vi "NTCP Read Msgs.vi"(5 "NTCP Read In":refnum<queue>, 7 "NTCP send in":refnum<queue>, 8 "error in (no error)":errorcluster, 11 "NTCP Actions":T4) -> (0 "error out":errorcluster, 1 "Targets":T2[](array[typedef]), 2 "Transaction ID":string, 3 "NTCP Status":T1, 4 "NTCP Read Out":refnum<queue>, 6 "NTCP send out":refnum<queue>)   [LabVIEW 2009]
uses:
  Launcher/Launcher Actions.ctl
  Launcher/NoPanelAppTypes.ctl
  Apps/App Status Actions.ctl
  NTCP library/NTCP Commands.ctl
  Data Access Objects/Metadata/LBCB Number.ctl
  MixedMode/Widget/Target.ctl
  NTCP Msg Types.ctl
  Global Data/Cartesian Measurment Actions.ctl
  NTCP Status.ctl
  Control Point Suffix.ctl
  NTCP library/Payload.ctl
  NTCP library/NTCP Message.ctl
  NTCP Client Actions.ctl
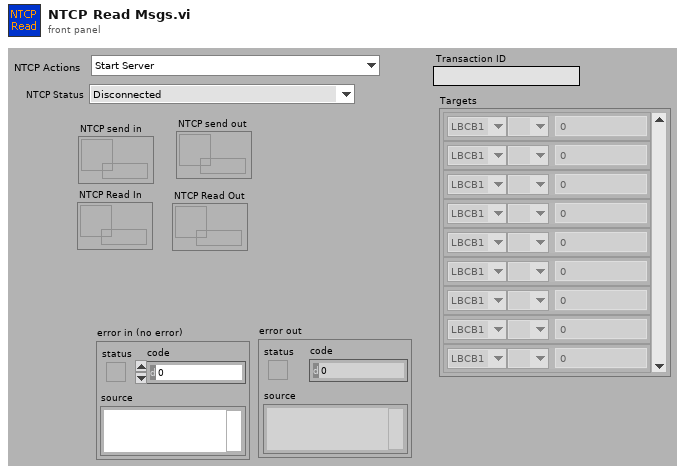
[diagram p1: front panel]
types:
  T1 = typedef "NTCP Status.ctl" = enum16{"Disconnected", "Connected", "Propose Targets Available", "Execute Requested"}
  T2 = typedef "Target.ctl" = cluster{"LBCB Number":T3, "DOF Vectors":enum16{" ", "Dx", "Dy", "Dz", "Rx", "Ry", "Rz", "Fx", "Fy", "Fz", "Mx", "My", "Mz"}, "Amount":dbl}
  T3 = typedef "LBCB Number.ctl" = enum16{"LBCB1", "LBCB2"}
  T4 = typedef "NTCP Client Actions.ctl" = enum16{"Start Server", "Listen", "Parse Message", "Shutdown Server"}
  T5 = typedef "App Status Actions.ctl" = enum16{"Init", "Get Status", "Running", "Control", "Autobalanced", "Data Acquisition", "Set App State", "DAQ Started", "Set LBCB State", "Set All", "Set Cont Logging", "Set Step Logging", "Set MM Logging", "Set Volt Logging", "Set Cart Type", "Set DAQ Link", "Set NTCP Link"}
  T6 = typedef "NoPanelAppTypes.ctl" = enum16{"NTCP Socket", "Data Archiving", "DAQ Link", "Control Loops", "Autobalance Monitor", "Mixed Mode Monitor", "Cart Plot", "Act Plot", "Cmd Disp Diffs"}
  T7 = typedef "Launcher Actions.ctl" = enum16{"Launch", "Stop All", "Stop", "Kill", "Running?", "Init"}
  T8 = typedef "NTCP Commands.ctl" = enum16{"propose", "execute", "cancel", "set-parameter", "get-parameter", "open-session", "close-session", "get-control-point", "Unknown", "stop"}
  T9 = typedef "NTCP Message.ctl" = cluster{"NTCP commands":T8, "Transaction ID":string, "Control Point":string, "Payload":T10[]}
  T10 = typedef "Payload.ctl" = cluster{"Content":string, "Control Point Suffix":T11}
  T11 = typedef "Control Point Suffix.ctl" = enum16{"LBCB1", "LBCB2", "ExternalSensors"}
  T12 = typedef "NTCP Msg Types.ctl" = enum16{"Control Point", "Step Done", "Propose Accepted", "Propose Not Accepted", "Propose Declined", "Propose Response", "Execute Done"}
  T13 = typedef "Cartesian Measurment Actions.ctl" = enum16{"Set Data", "Get", "Init", "Set Offsets"}
  T14 = typedef "Propose Command.ctl" = cluster{"Control Type":i32[], "Value":dbl[]}
  T15 = typedef "App Status.ctl" = cluster{"Running":bool, "Controlling L2":bool, "Autobalance L2":bool, "Data Acquisition":bool, " App State":T16, "DAQ Started":bool, "LBCB 1 State":T17, "LBCB 2 State":T17, "Controlling L1":bool, "Autobalance L1":bool, "Cartesian Type":bool, "Continuous Logging":bool, "Step Logging":bool, "Voltage Logging":bool, "Mixed Mode Logging":bool, "DAQ Link":bool, "NTCP Link ":bool}
  T16 = typedef "AppStates.ctl" = enum16{"Starting OM", "Initializing Displays", "Setting up Archiving", "Setting Up DAQ Channels", "Start DAQ", "DAQ Starting", "Controlling LBCBs", "Stopping OM"}
  T17 = typedef "Lbcb Control Loop States.ctl" = enum16{"Idle", "Start Selected", "Load Last Command", "Start Autobalancing", "Autobalancing", "Control Loop Initialized", "Control Enabled"}
  T18 = typedef "Cartesian Data Type.ctl" = cluster{"Displacements":dbl[], "Forces":dbl[], "Displacement Commands":dbl[]}
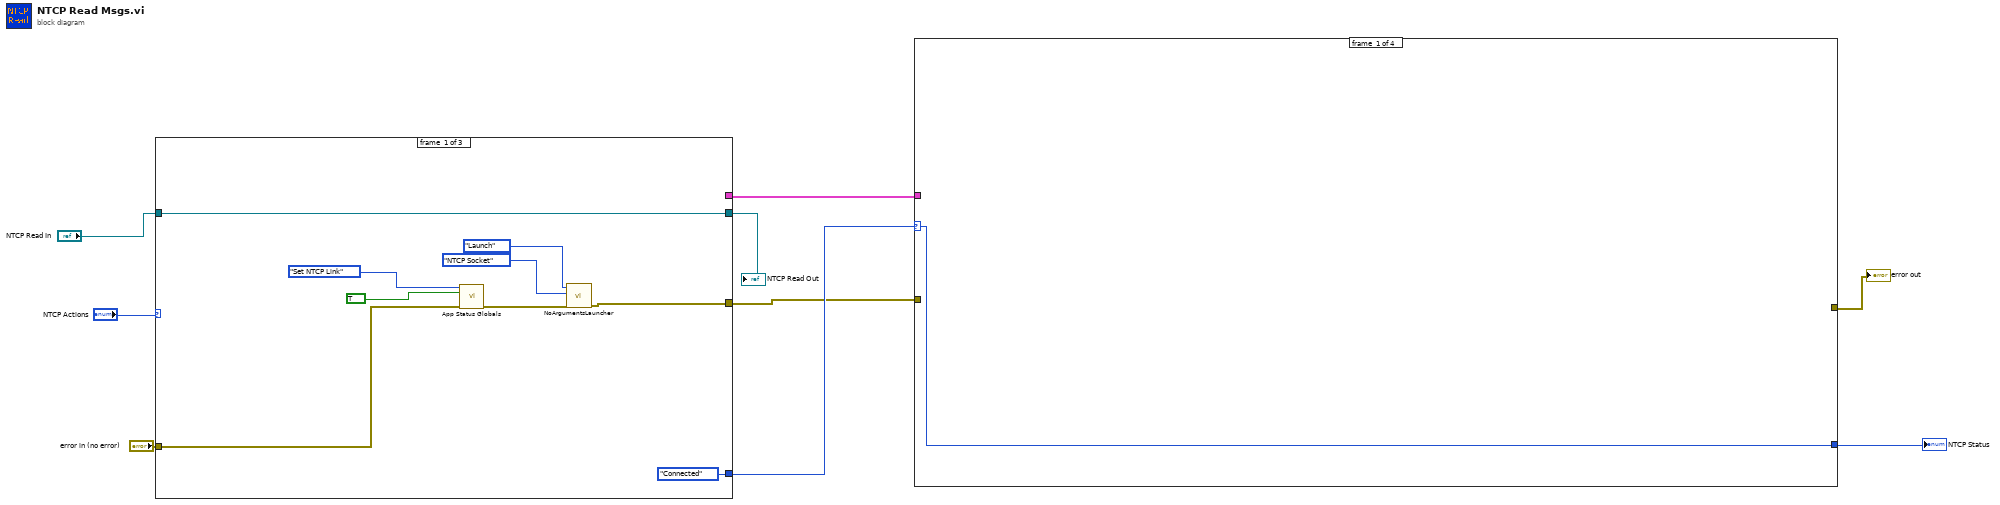
[diagram p0: block diagram]
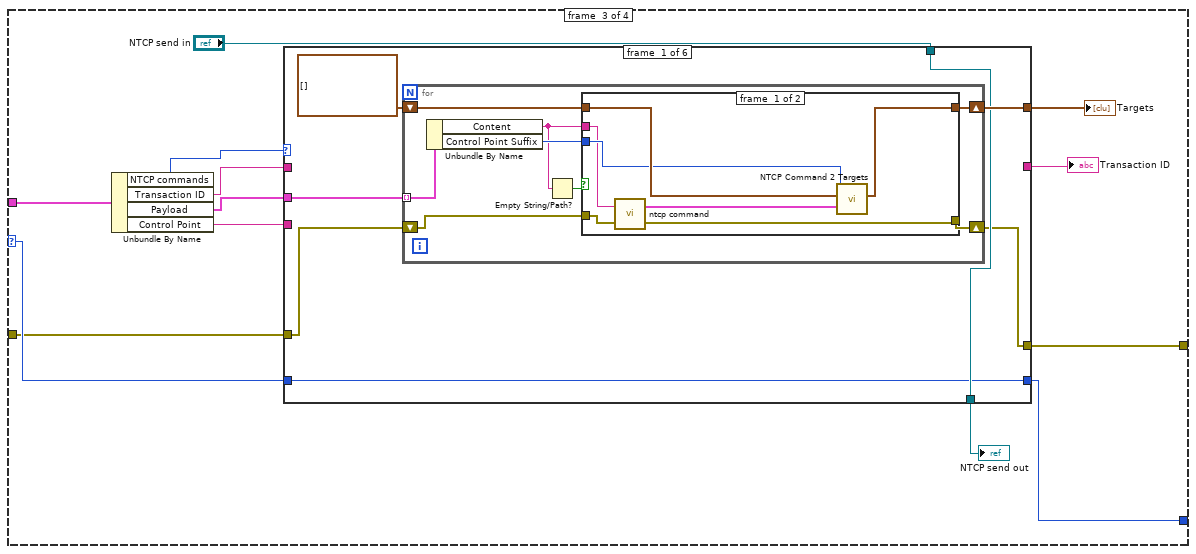
[diagram p3: hidden frame]
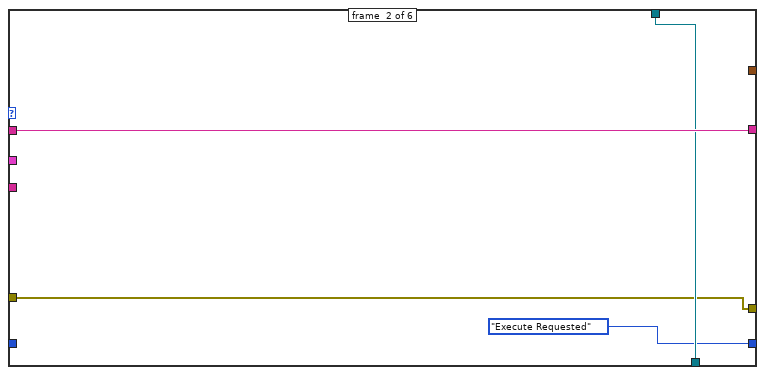
[diagram p5: hidden frame]
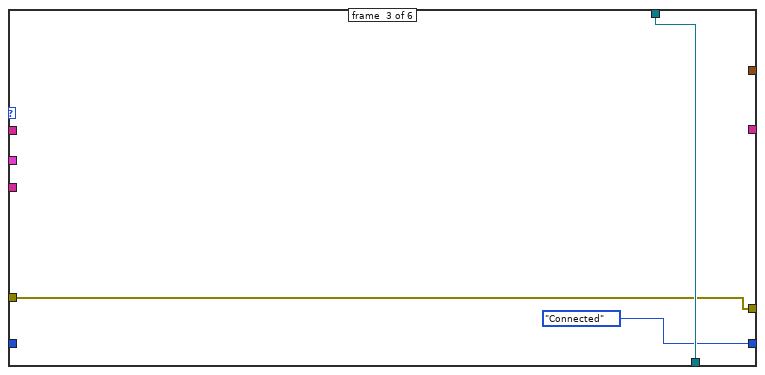
[diagram p6: hidden frame]
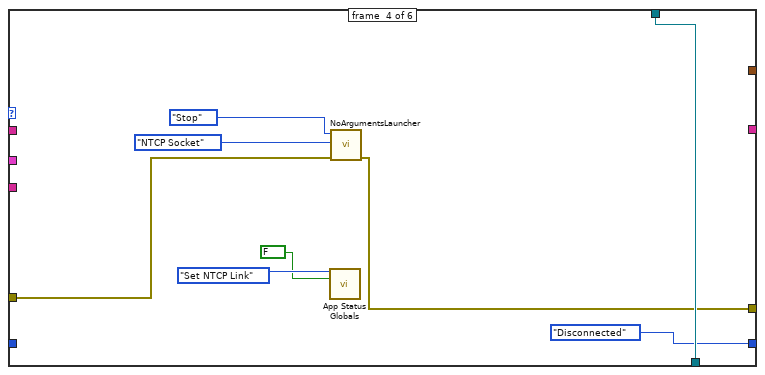
[diagram p7: hidden frame]
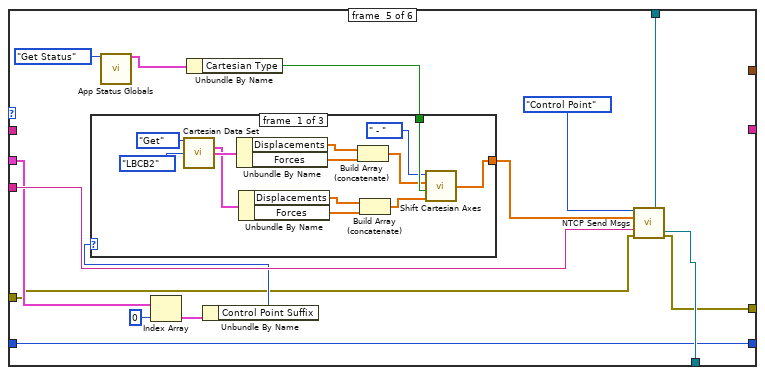
[diagram p8: hidden frame]
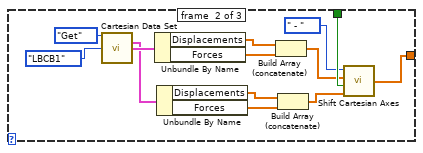
[diagram p9: hidden frame]
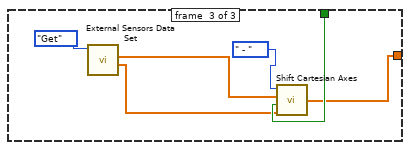
[diagram p10: hidden frame]
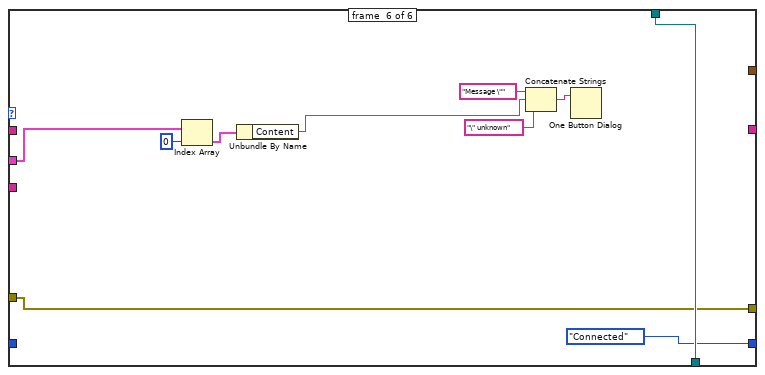
[diagram p11: hidden frame]
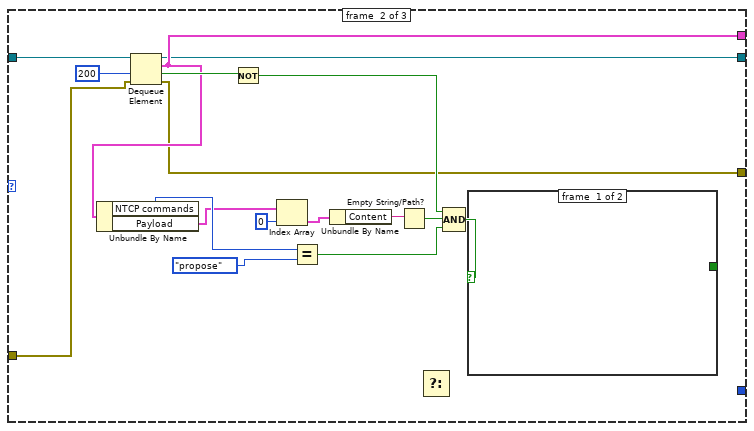
[diagram p13: hidden frame]
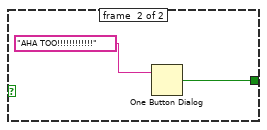
[diagram p14: hidden frame]
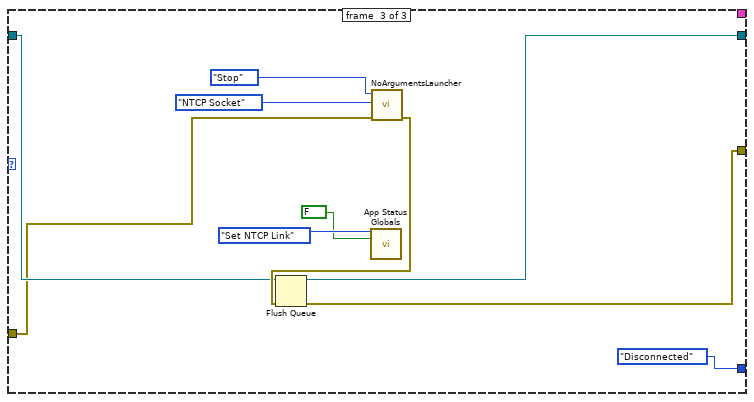
[diagram p15: hidden frame]
diagram:
  n1 = case shown="\"Shutdown Server\"" "NTCP Actions" {
    tunnel: [w13 w21 w39] -> w2
    tunnel: "error in (no error)" -> [w12 w22 w40]
    tunnel: [_ w23 _] -> w5
    tunnel: "NTCP Read In" -> [w10 w20 w42]
    tunnel: [w10 w19 w41] -> w6
    tunnel: [NTCP_Status."Connected" ("NTCP Status") _ NTCP_Status."Disconnected" ("NTCP Status")] -> w4
    frame #0 {
      n2 = call "App Status Globals.vi"("App Status Actions"=App_Status_Actions."Set NTCP Link", "Status\nSetting"=TRUE ("Status\nSetting"), "error in (no error)"=w12) -> ("error out"=w16:errorcluster)  [unwired: 11 in, 1 out]
      n3 = call "NoArgumentsLauncher.vi"("error in (no error)"=w16, "Application"=NoPanelAppTypes."NTCP Socket", "Application Launcher Actions"=Launcher_Actions."Launch") -> ("error out"=w13:errorcluster)  [unwired: 8 out]
    }
    frame #1 {
      n4 = Dequeue Element(queue=w20, timeout in ms (-1)=200, error in (no error)=w22) -> (queue out=w19:refnum<queue>, element=w23:T9, timed out?=w32:bool, error out=w21:errorcluster)
      n5 = Unbundle By Name(w23) -> ("NTCP commands"=w34:T8, "Payload"=w33:T10[])
      n6 = Not(x=w32) -> (.not. x?=w35:bool)
      n7 = Index Array(array=w33, index=0) -> (element=w29:T10)
      n8 = Equal?(x=w34, y=NTCP_Commands."propose" ("NTCP commands")) -> (x = y?=w26:bool)
      n9 = Unbundle By Name(w29) -> ("Content"=w28:string)
      n10 = Empty String/Path?(string/path=w28) -> (empty?=w27:bool)
      n11 = Select() -> ()  [unwired: 3 in, 1 out]
      n12 = Compound Arithmetic op=AND(w35, w27, w26) -> (w25:bool)
      n13 = case shown="True" w25 {
        tunnel: [_ w36] -> _
        frame #0 {
        }
        frame #1 {
          n14 = One Button Dialog(message="AHA TOO!!!!!!!!!!!!") -> (true=w36:bool)  [unwired: 1 out]
        }
      }
    }
    frame #2 {
      n15 = call "App Status Globals.vi"("App Status Actions"=App_Status_Actions."Set NTCP Link", "Status\nSetting"=FALSE ("Execute Pending")) -> ()  [unwired: 12 in, 2 out]
      n16 = call "NoArgumentsLauncher.vi"("error in (no error)"=w40, "Application"=NoPanelAppTypes."NTCP Socket", "Application Launcher Actions"=Launcher_Actions."Stop") -> ("error out"=w45:errorcluster)  [unwired: 8 out]
      n17 = Flush Queue(queue=w42, error in (no error)=w45) -> (queue out=w41:refnum<queue>, error out=w39:errorcluster)  [unwired: 1 out]
    }
  }
  "NTCP Read Out" <- w6
  n18 = case shown="\"Propose Targets Available\"" w4 {
    selector: w4 -> [w48 _ w52 _]
    tunnel: w5 -> [_ _ w61 _]
    tunnel: [w48 _ w51 _] -> w3
    tunnel: w2 -> [_ _ w50 _]
    tunnel: [_ _ w49 _] -> w1
    frame #0 {
    }
    frame #1 {
    }
    frame #2 {
      n19 = Unbundle By Name(w61) -> ("NTCP commands"=w60:T8, "Transaction ID"=w58:string, "Payload"=w59:T10[], "Control Point"=w57:string)
      n20 = case shown="\"Unknown\"" w60 {
        tunnel: w59 -> [w68 _ _ _ w105 w150]
        tunnel: [w66 _ _ _ _ _] -> w53
        tunnel: [_ w89 _ _ _ _] -> w54
        tunnel: w58 -> [_ w89 _ _ _ _]
        tunnel: w57 -> [_ _ _ _ w110 _]
        tunnel: "NTCP send in" -> [w65 w88 w92 w100 w109 w157]
        tunnel: [w65 w88 w92 w100 w108 w157] -> w55
        tunnel: w52 -> [w64 _ _ _ w103 _]
        tunnel: [w64 NTCP_Status."Execute Requested" ("NTCP Status") NTCP_Status."Connected" ("NTCP Status") NTCP_Status."Disconnected" ("NTCP Status") w103 NTCP_Status."Connected" ("NTCP Status")] -> w51
        tunnel: w50 -> [w63 w86 w90 w94 w102 w149]
        tunnel: [w62 w86 w90 w93 w101 w149] -> w49
        frame #0 {
          n21 = for {
            shift-right: [w75] -> w66
            shift-left: T2[] [] ("Step Out") -> [w76]
            tunnel: w68 -> [w74] mode=indexing
            shift-right: [w69] -> w62
            shift-left: w63 -> [w70]
            n22 = Unbundle By Name(w74) -> ("Content"=w71:string, "Control Point Suffix"=w73:T11)
            n23 = Empty String/Path?(string/path=w71) -> (empty?=w72:bool)
            n24 = case shown="True" w72 {
              tunnel: w76 -> [w82 w85]
              tunnel: [w79 w85] -> w75
              tunnel: w73 -> [w81 _]
              tunnel: w71 -> [w80 _]
              tunnel: w70 -> [w78 w84]
              tunnel: [w77 w84] -> w69
              frame #0 {
                n25 = call "ntcp command.vi"("error in"=w78, "Input string"=w80) -> ("Error out"=w77:errorcluster, "NTCP Command"=w83:T14)
                n26 = call "NTCP Command 2 Targets.vi"("NTCP Command"=w83, "Targets In"=w82, "Contol\nPoint\nSuffix"=w81) -> ("Targets Out"=w79:T2[])  [unwired: 8 out]
              }
              frame #1 {
              }
            }
          }
        }
        frame #1 {
        }
        frame #2 {
        }
        frame #3 {
          n27 = call "App Status Globals.vi"("App Status Actions"=App_Status_Actions."Set NTCP Link", "Status\nSetting"=FALSE ("Execute Pending")) -> ()  [unwired: 12 in, 2 out]
          n28 = call "NoArgumentsLauncher.vi"("error in (no error)"=w94, "Application"=NoPanelAppTypes."NTCP Socket", "Application Launcher Actions"=Launcher_Actions."Stop") -> ("error out"=w93:errorcluster)  [unwired: 8 out]
        }
        frame #4 {
          n29 = call "App Status Globals.vi"("App Status Actions"=App_Status_Actions."Get Status") -> ("App Status Out"=w114:T15)  [unwired: 5 in, 9 out]
          n30 = Index Array(array=w105, index=0) -> (element=w106:T10)
          n31 = Unbundle By Name(w114) -> ("Cartesian Type"=w115:bool)
          n32 = Unbundle By Name(w106) -> ("Control Point Suffix"=w104:T11)
          n33 = case shown="\"LBCB2\"" w104 {
            tunnel: [w116 w129 w142] -> w112
            tunnel: w115 -> [w120 w133 w145]
            frame #0 {
              n34 = call "Cartesian Data Set.vi"("Measurement Actions"=Cartesian_Measurment_Actions."Get", "LBCB Selected"=LBCB_Number."LBCB2") -> ("Cartesian Data Offsets Out"=w121:T18, "Cartesian Data Hold Data Out"=w126:T18)  [unwired: 4 in, 8 out]
              n35 = Unbundle By Name(w126) -> ("Displacements"=w125:dbl[], "Forces"=w124:dbl[])
              n36 = Unbundle By Name(w121) -> ("Displacements"=w122:dbl[], "Forces"=w123:dbl[])
              n37 = Build Array (concatenate)(w125, w124) -> (w117:dbl[])
              n38 = Build Array (concatenate)(w122, w123) -> (w118:dbl[])
              n39 = call "Shift Cartesian Axes.vi"("Coordianate Offset"=w118, "Coordinate Switch"=w120, "Coordianate Input"=w117, "Direction"=enum16{" +", " - "}." - ") -> ("Coordianate Output"=w116:dbl[])
            }
            frame #1 {
              n40 = call "Cartesian Data Set.vi"("Measurement Actions"=Cartesian_Measurment_Actions."Get", "LBCB Selected"=LBCB_Number."LBCB1") -> ("Cartesian Data Offsets Out"=w134:T18, "Cartesian Data Hold Data Out"=w139:T18)  [unwired: 4 in, 8 out]
              n41 = Unbundle By Name(w139) -> ("Displacements"=w138:dbl[], "Forces"=w137:dbl[])
              n42 = Unbundle By Name(w134) -> ("Displacements"=w135:dbl[], "Forces"=w136:dbl[])
              n43 = Build Array (concatenate)(w138, w137) -> (w130:dbl[])
              n44 = Build Array (concatenate)(w135, w136) -> (w131:dbl[])
              n45 = call "Shift Cartesian Axes.vi"("Coordianate Offset"=w131, "Coordinate Switch"=w133, "Coordianate Input"=w130, "Direction"=enum16{" +", " - "}." - ") -> ("Coordianate Output"=w129:dbl[])
            }
            frame #2 {
              n46 = call "External Sensors Data Set.vi"("Measurement Actions"=Cartesian_Measurment_Actions."Get") -> ("Offsets"=w143:dbl[], "Hold Data Out"=w144:dbl[])  [unwired: 3 in, 6 out]
              n47 = call "Shift Cartesian Axes.vi"("Coordianate Offset"=w143, "Coordinate Switch"=w145, "Coordianate Input"=w144, "Direction"=enum16{" +", " - "}." - ") -> ("Coordianate Output"=w142:dbl[])
            }
          }
          n48 = call "NTCP Send Msgs.vi"("Message Type"=NTCP_Msg_Types."Control Point", "queue in"=w109, "Hold Data"=w112, "ControlPoint name"=w110, "error in (no error)"=w102) -> ("queue out"=w108:refnum<queue>, "error out"=w101:errorcluster)  [unwired: 3 in, 6 out]
        }
        frame #5 {
          n49 = Index Array(array=w150, index=0) -> (element=w155:T10)
          n50 = Unbundle By Name(w155) -> ("Content"=w156:string)
          n51 = Concatenate Strings("Message \"" ("string"), w156, "\" unknown" ("string")) -> (w151:string)
          n52 = One Button Dialog(message=w151) -> ()  [unwired: 2 out]
        }
      }
      "NTCP send out" <- w55
      "Targets" <- w53
      "Transaction ID" <- w54
    }
    frame #3 {
    }
  }
  "error out" <- w1
  "NTCP Status" <- w3
